vi "Test Launcher.vi"() -> ()   [LabVIEW 2017, in "Test Actor.lvclass"]
doc: "Launches several test actors to display the monitored actor window\n\nCopyright: MGI\nAuthored by: Derek Trepanier"
uses:
  Test Actor.lvclass
  C:/Program Files (x86)/National Instruments/LabVIEW 2017/vi.lib/ActorFramework/Actor/Actor.lvclass
  Test Actor.lvclass/Test Actor.ctl
  <vilib>/ActorFramework/Message Queue/Message Queue.lvclass/Message Queue.ctl
  <vilib>/ActorFramework/Message Enqueuer/Message Enqueuer.lvclass/Message Enqueuer.ctl
  <vilib>/ActorFramework/Message Enqueuer/Enqueue.vi
  <vilib>/ActorFramework/Stop Msg/Stop Msg.lvclass
  C:/Program Files (x86)/National Instruments/LabVIEW 2017/vi.lib/ActorFramework/Message/Message.lvclass
  <vilib>/ActorFramework/Message Priority Queue/Priority Enqueue.vi
  <vilib>/ActorFramework/Actor/Actor.lvclass
  <vilib>/ActorFramework/Message Queue/Message Queue.lvclass
panel:
  in  "stop":bool
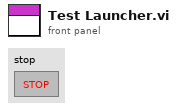
[diagram p1: front panel]
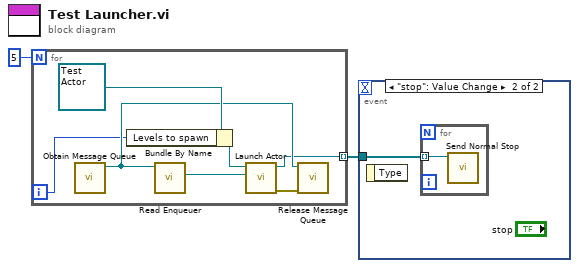
[diagram p0: block diagram]
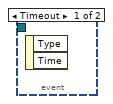
[diagram p2: hidden frame]
diagram:
  n1 = for {
    N: 5 -> [_]
    tunnel: [w4] -> w1 mode=indexing
    i -> [w3]
    n2 = call <vilib>:"Obtain Message Queue.vi"() -> ("Message Queue"=w7:refnum<class "Message Queue.lvclass">)  [unwired: 10 in, 1 out]
    n3 = Bundle By Name(cluster=refnum<class "Test Actor.lvclass"> refnum ("Test Actor.lvclass"), "Levels to spawn"=w3) -> (w5:refnum<class "Test Actor.lvclass">)
    n4 = call <vilib>:"Read Enqueuer.vi"("Message Queue"=w7) -> ("Message Enqueuer"=w9:refnum<class "Message Enqueuer.lvclass">)  [unwired: 10 in]
    n5 = call <vilib>:"Launch Actor.vi"("Actor-to-Caller Enqueuer"=w9, "Actor"=w5) -> ("error out"=w6:errorcluster, "Caller-To-Actor Enqueuer"=w4:refnum<class "Message Enqueuer.lvclass">)  [unwired: 8 in]
    n6 = call <vilib>:"Release Message Queue.vi"("error in (no error)"=w6, "Message Queue"=w7) -> ()  [unwired: 8 in, 2 out]
  }
  n7 = event shown="[1] \"stop\": Value Change" {
    selector: _ -> [_ _]
    dyn-events: _ -> [_ _]
    timeout: _ -> [_ _]
    tunnel: w1 -> [_ w10]
    event Timeout {
      n8 = event-data() -> ()  [unwired: 1 in, 2 out]
    }
    event "stop": Value Change {
      n9 = event-data() -> ()  [unwired: 1 in, 1 out]
      n10 = for {
        tunnel: w10 -> [w11] mode=indexing
        n11 = call <vilib>:"Send Normal Stop.vi"("Message Enqueuer"=w11) -> ()  [unwired: 10 in, 1 out]
      }
    }
  }
